vi "Write File Location.vi"(8 "error in (no error)":errorcluster, 10 "File Location":path, 11 "UserPreferencesFileManager in":refnum<class "User Preferences File.lvclass">) -> (0 "error out":errorcluster, 3 "UserPreferencesFileManager out":refnum<class "User Preferences File.lvclass">)   [LabVIEW 2020, in "RxnRover.lvlib" / "User Preferences File.lvclass"]
uses:
  User Preferences File.lvclass
  User Preferences File.lvclass/User Preferences File.ctl
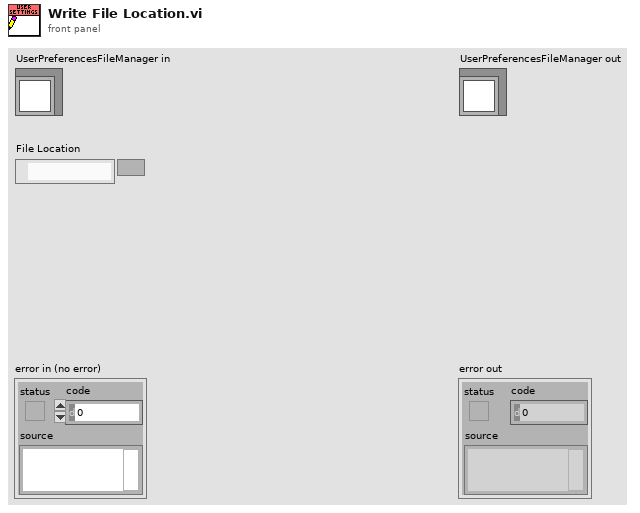
[diagram p1: front panel]
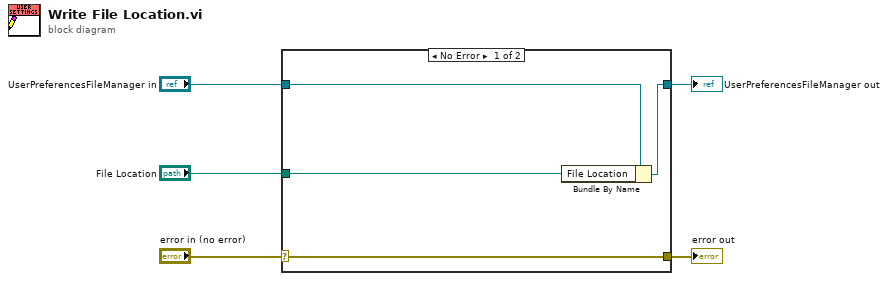
[diagram p0: block diagram]
diagram:
  n1 = case shown="No Error" "error in (no error)" {
    selector: "error in (no error)" -> [w9 w10]
    tunnel: [w9 w10] -> w4
    tunnel: [w7 w11] -> w2
    tunnel: "UserPreferencesFileManager in" -> [w8 w11]
    tunnel: "File Location" -> [w6 _]
    frame No Error {
      n2 = Bundle By Name(cluster=w8, "File Location"=w6) -> (w7:refnum<class "User Preferences File.lvclass">)
    }
    frame Error {
    }
  }
  "error out" <- w4
  "UserPreferencesFileManager out" <- w2
